vi "myRIO_BRig_FPGA_v3,31__PortC.vi"() -> ()   [LabVIEW 2014]
uses:
  <vilib>/rvi/FXPMathLib/FxpDiv/subVIs/nifxpmath_Div_SimConfig.ctl
  <vilib>/rvi/FXPMathLib/FxpSinAndCos/subVIs/nifxpmath_SinAndCos_SimConfig.ctl
  <vilib>/rvi/FXPMathLib/FxpDiv/simVIs/DllFxpDivTemp_sub.vi
  <vilib>/rvi/FXPMathLib/FxpSinAndCos/simVIs/DllFxpSinAndCosTemp_sub.vi
  <vilib>/rvi/Emulation/niFpgaGetClockAttributes.vi
  <vilib>/rvi/Emulation/niFpgaSctlEmulationGetInTimedLoop.vi
  <vilib>/rvi/Emulation/niFpgaEmulationReportErrorSimple.vi
  <vilib>/rvi/eio/common/nirviEmuTemplateMethod_errors.vi
  <vilib>/rvi/Emulation/niFpgaCriticalErrorInLSC.vi
  <vilib>/rvi/FXPMathLib/FxpDiv/XNode/nifxpmath_Div.xnode
  <vilib>/rvi/FXPMathLib/FxpMul/XNode/nifxpmath_Multiplier.xnode
  <vilib>/rvi/FXPMathLib/FxpSinAndCos/XNode/nifxpmath_SinAndCos.xnode
  <vilib>/rvi/FXPMathLib/FxpSub/XNode/nifxpmath_Sub.xnode
  <vilib>/eio/EIONode/EIONode.xnode
  <vilib>/rvi/FXPMathLib/sim/FxpSim.dll
panel:
  in  "laser_Nshutter":u32=100
  in  "AnaOut_0":i16
  in  "f_time_select":u32=173
  in  "laser_Nvalley":u32=100
  in  "laser_Npeak":u32=100
  in  "laserledMTrig":bool
  in  "tCycle_laser_wro":u32=100
  in  "tDelay_laser_wro":u32
  in  "tCycle_laser_rew":u32=100
  in  "tDelay_laser_rew":u32
  in  "laserResponse_reward_LED":bool
  in  "laserResponse_wrong_LED":bool
  out "SelectWrong":bool
  out "SelectReward":bool
  in  "laserResponse_wrong":bool
  in  "laserResponse_reward":bool
  in  "Left(F)_or_Right(T)":bool
  in  "ignoreWrong":bool
  in  "SelectionState":bool
  in  "laserMTrig":bool
  in  "FPGA_Stop":bool
  in  "audioTrigger_L":bool
  in  "audioTrigger_R":bool
  in  "audioFreq_L_Hz":u16=1000 min=1000 max=14000 step=1000
  in  "audioAmp_L":u16=1 min=1 max=32767 step=1
  in  "audioFreq_R_Hz":u16=1000 min=1000 max=14000 step=1000
  in  "audioAmp_R":u16=1 min=1 max=32767 step=1
  in  "A3_SL":bool
  in  "A1_SR":bool
  in  "Counts_Reset":bool
  out "A4_LickR":u32
  out "A2_LickL":u32
  in  "A6_Act":bool
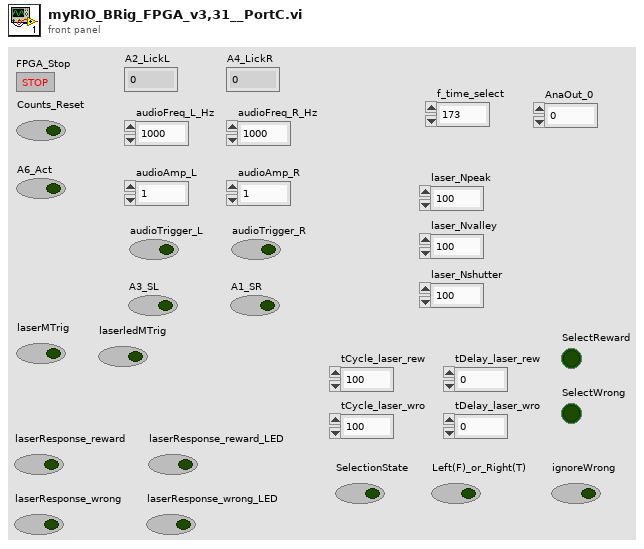
[diagram p1: front panel]
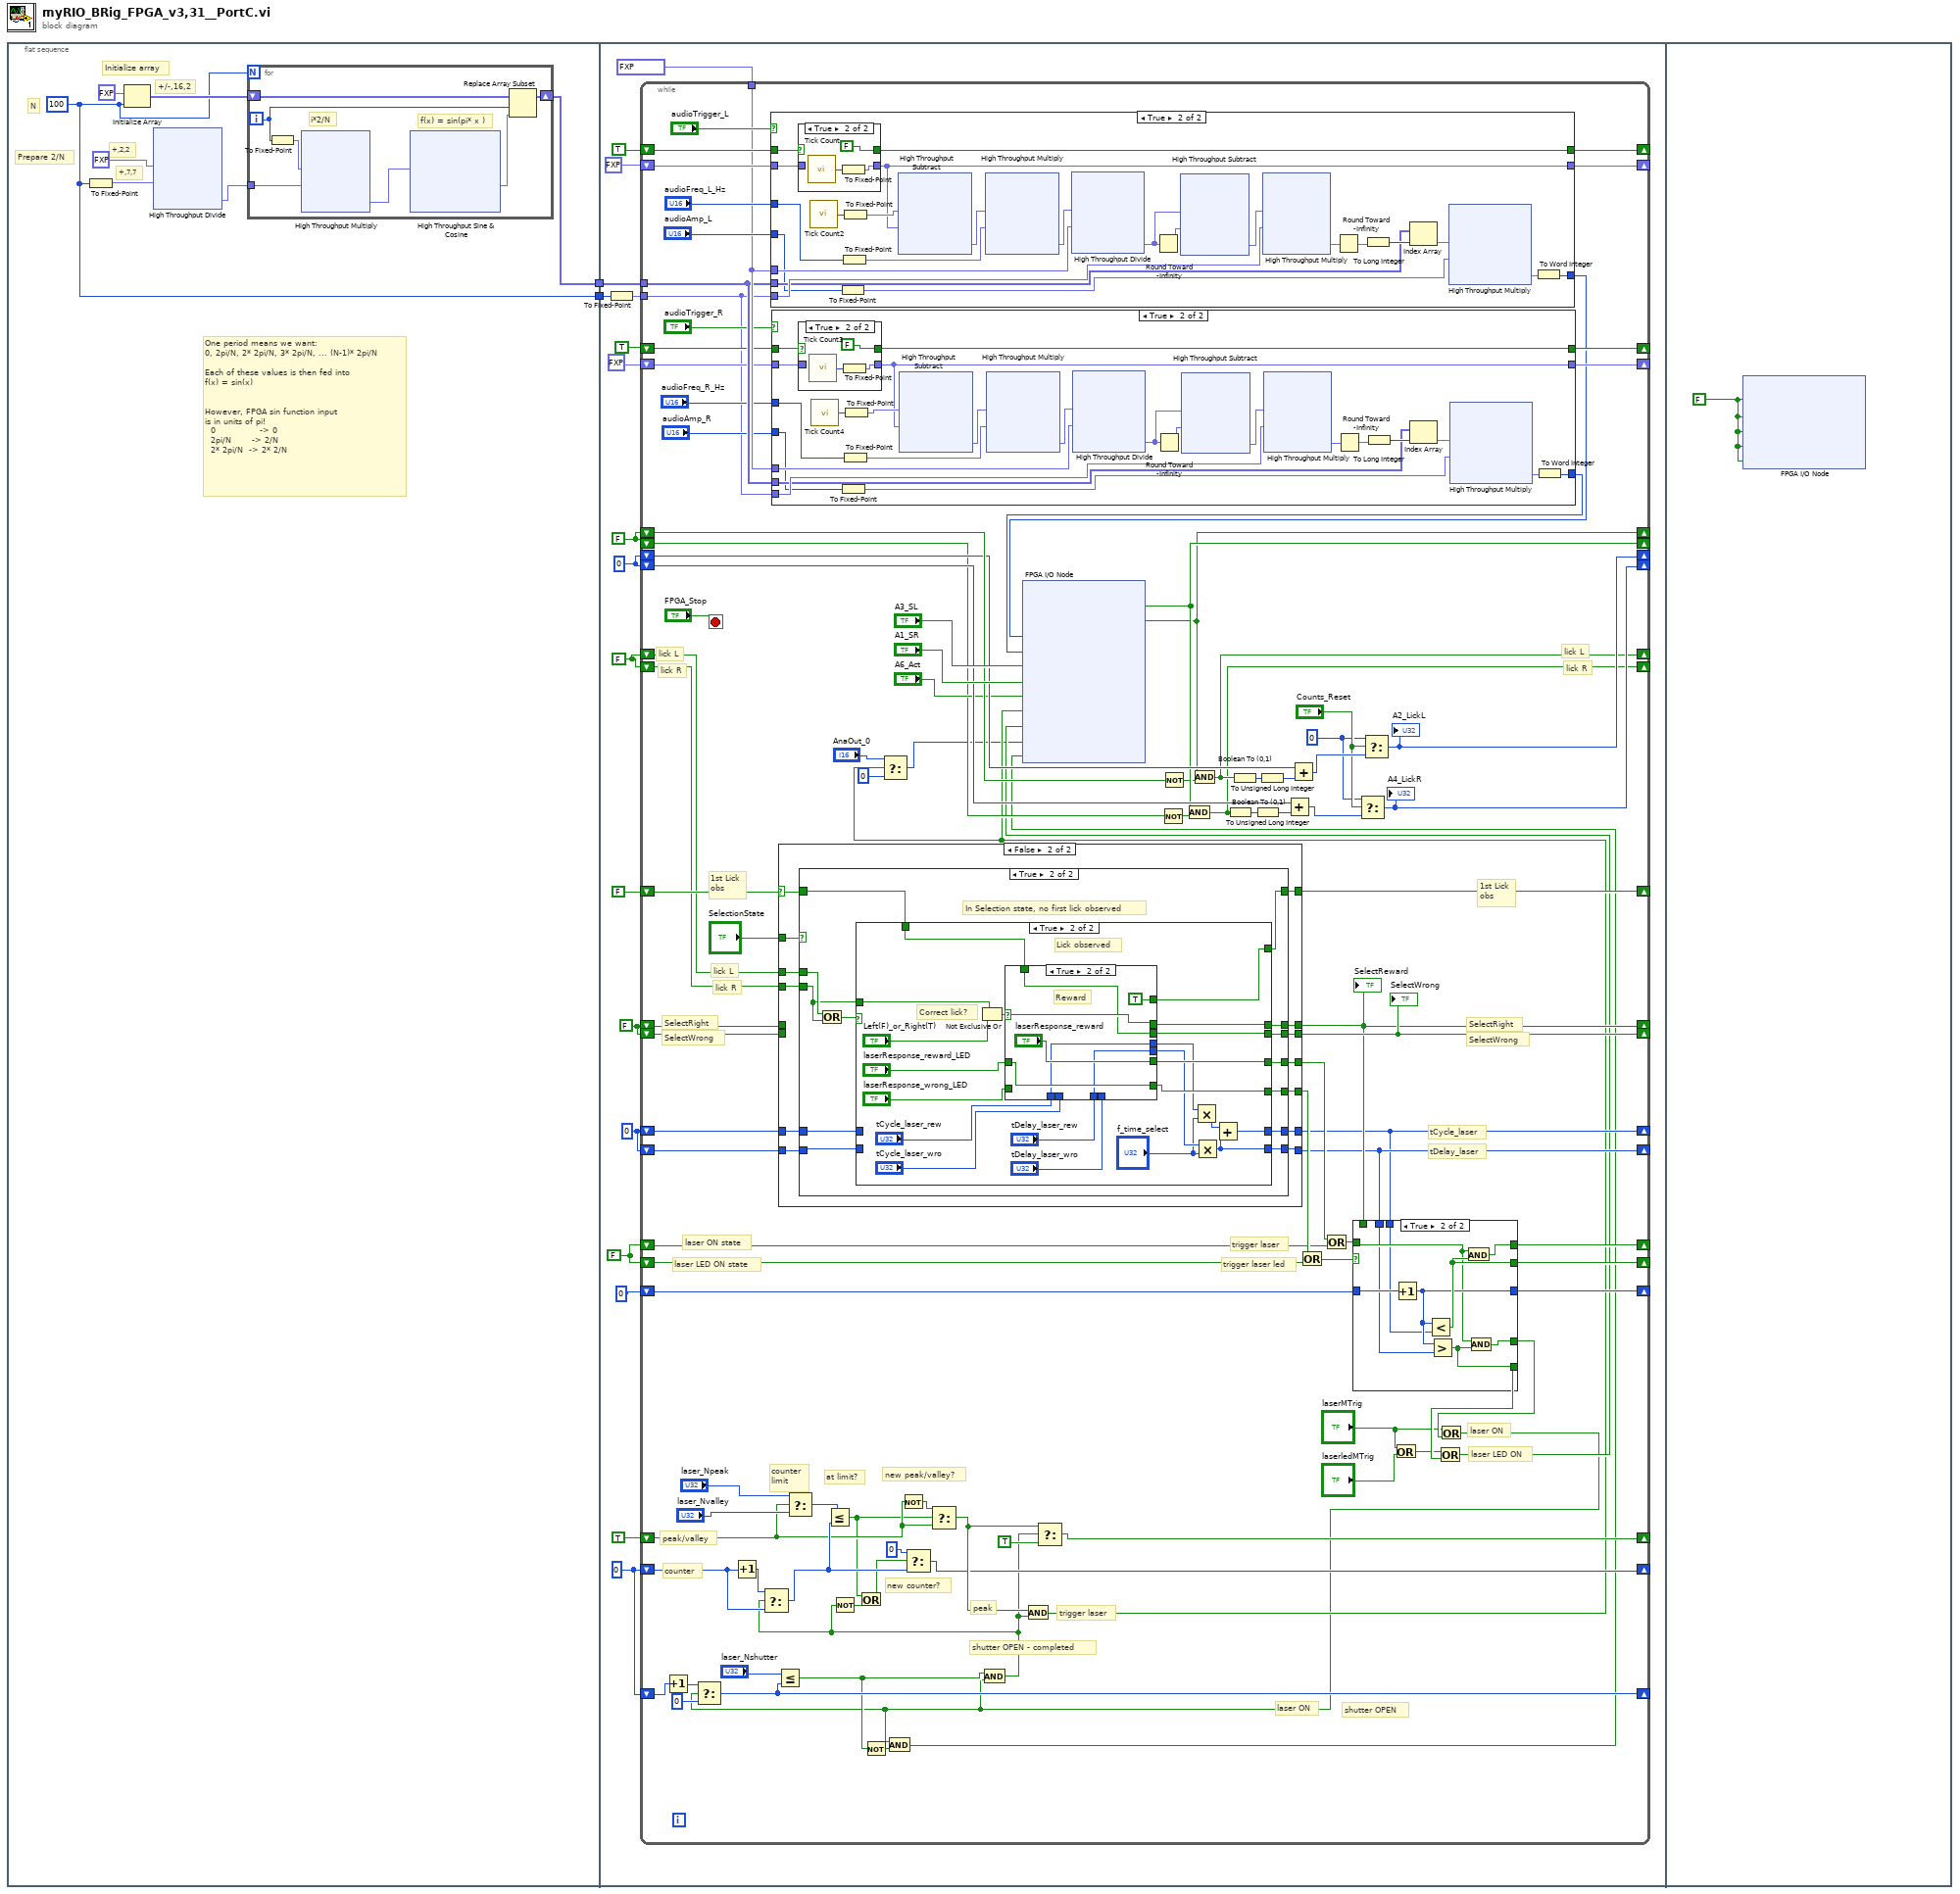
[diagram p0: block diagram]
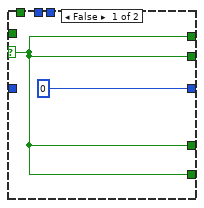
[diagram p2: hidden frame]
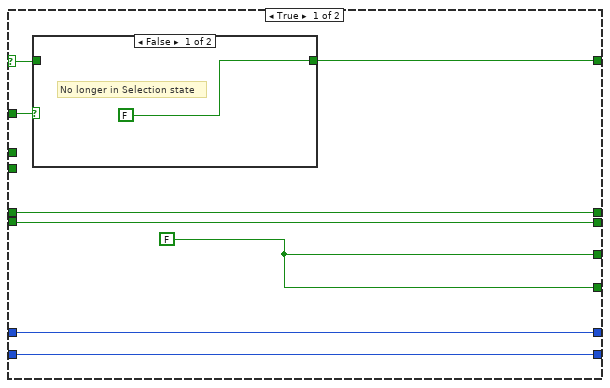
[diagram p3: hidden frame]
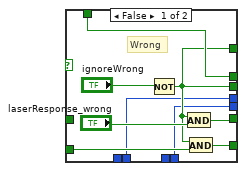
[diagram p7: hidden frame]
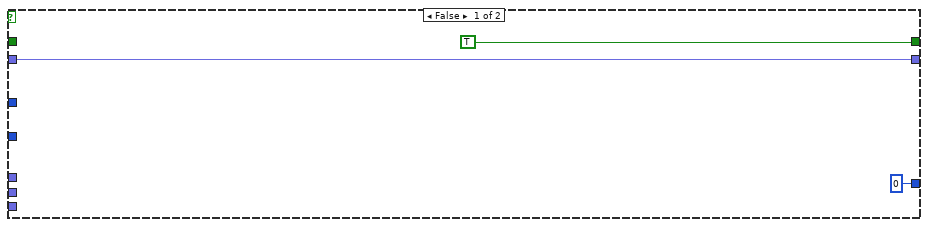
[diagram p8: hidden frame]
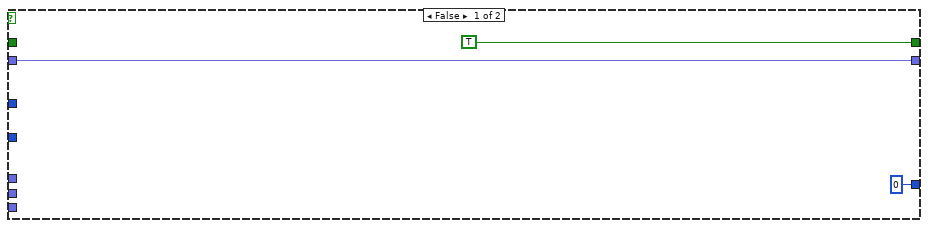
[diagram p10: hidden frame]
diagram:
  n1 = flat-sequence {
    tunnel: [w4] -> w2
    tunnel: [w3] -> w1
    tunnel: w2 -> [w86]
    tunnel: w1 -> [w88]
    frame #0 {
      w3 = 100 ("dimension size")
      # "N"
      # "+,7,7"
      # "+,2,2"
      # "+/-,16,2"
      # "Prepare 2/N"
      # "One period means we want:\n0, 2pi/N, 2* 2pi/N, 3* 2pi/N, ... (N-1)* 2pi/N\n\nEach of these values is then fed into\nf(x) = sin(x)\n\n\nHowever, FPGA sin function input\nis in units of pi!\n  0               -> 0\n  2pi/N       -> 2/N\n  2* 2pi/N  -> 2* 2/N"
      # "Initialize array"
      n2 = To Fixed-Point(number=w3) -> (fixed-point=w6:fxp<+,7,7>)  [unwired: 1 in]
      n3 = Initialize Array(fxp<+/-,16,2> 0.0 ("element"), w3) -> (w9:fxp<+/-,16,2>[])
      n4 = xnode "High Throughput Divide"("x"=fxp<+,2,2> 2.0, "y"=w6) -> ("x/y"=w5:fxp<+,27,0>)
      n5 = for {
        N: w3 -> [_]
        shift-right: [w42] -> w4
        shift-left: w9 -> [w43]
        tunnel: w5 -> [w38]
        i -> [w41]
        # "f(x) = sin(pi* x )"
        # "i*2/N"
        n6 = To Fixed-Point(number=w41) -> (fixed-point=w39:fxp<+,7,7>)  [unwired: 1 in]
        n7 = xnode ("High Throughput Multiply")("x"=w39, "y"=w38) -> ("x*y"=w37:fxp<+,34,7>)
        n8 = xnode "High Throughput Sine & Cosine"("x (pi)"=w37) -> ("sin(x)"=w40:fxp<+/-,16,2>)  [unwired: 1 out]
        n9 = Replace Array Subset(array=w43, new element=w40, index=w41) -> (w42:fxp<+/-,16,2>[])
      }
    }
    frame #1 {
      w74 = u32 0
      w76 = u32 0
      w78 = FALSE
      w77 = FALSE
      w81 = FALSE
      w82 = FALSE
      w83 = u32 0
      n10 = To Fixed-Point(number=w88) -> (fixed-point=w87:fxp<+,7,7>)  [unwired: 1 in]
      n11 = while {
        shift-right: [w187] -> _
        shift-left: TRUE -> [w191]
        shift-right: [w186] -> _
        shift-left: fxp<+,32,32> 0.0 -> [w190]
        tunnel: fxp<+,17,26> 40000000.0 -> [w185]
        tunnel: w87 -> [w178]
        tunnel: w86 -> [w184]
        shift-right: [w177] -> _
        shift-left: TRUE -> [w183]
        shift-right: [w176] -> _
        shift-left: fxp<+,32,32> 0.0 -> [w182]
        shift-right: [w153] -> _
        shift-left: w83 -> [w165]
        shift-right: [w156] -> _
        shift-left: w83 -> [w169]
        shift-right: [w157] -> _
        shift-left: w82 -> [w160]
        shift-right: [w154] -> _
        shift-left: w82 -> [w166]
        shift-right: [w151] -> _
        shift-left: FALSE -> [w150]
        shift-right: [w149] -> _
        shift-left: w81 -> [w147]
        shift-right: [w148] -> _
        shift-left: w81 -> [w146]
        shift-right: [w136] -> _
        shift-left: w77 -> [w138]
        shift-right: [w144] -> _
        shift-left: u32 0 -> [w145]
        shift-right: [w130] -> _
        shift-left: w78 -> [w142]
        shift-right: [w143] -> _
        shift-left: w78 -> [w141]
        shift-right: [w137] -> _
        shift-left: w77 -> [w134]
        shift-right: [w126] -> _
        shift-left: w76 -> [w129]
        shift-right: [w127] -> _
        shift-left: w76 -> [w128]
        shift-right: [w109] -> _
        shift-left: w74 -> [w120]
        shift-right: [w110] -> _
        shift-left: TRUE -> [w113]
        shift-right: [w97] -> _
        shift-left: w74 -> [w101]
        stop <- "FPGA_Stop" stop-if-true
        w162 = u32 0
        # "shutter OPEN"
        # "shutter OPEN - completed"
        # "trigger laser"
        # "peak"
        # "laser ON"
        # "new peak/valley?"
        # "counter"
        # "peak/valley"
        # "new counter?"
        # "at limit?"
        # "counter\nlimit"
        # "tDelay_laser"
        # "tCycle_laser"
        # "laser LED ON"
        # "laser ON"
        # "laser LED ON state"
        # "laser ON state"
        # "SelectWrong"
        # "SelectRight"
        # "SelectWrong"
        # "SelectRight"
        # "lick R"
        # "lick L"
        # "1st Lick\nobs"
        # "1st Lick\nobs"
        # "lick R"
        # "lick L"
        # "lick R"
        # "lick L"
        # "trigger laser led"
        # "trigger laser"
        n12 = Increment(x=w101) -> (x+1=w100:u32)
        n13 = Increment(x=w120) -> (x+1=w118:u32)
        n14 = case shown="True" "audioTrigger_L" {
          tunnel: w191 -> [_ w369]
          tunnel: w190 -> [w345 w368]
          tunnel: "audioFreq_L_Hz" -> [_ w365]
          tunnel: w185 -> [_ w362]
          tunnel: [w345 w346] -> w186
          tunnel: [TRUE w359] -> w187
          tunnel: w178 -> [_ w358]
          tunnel: w184 -> [_ w353]
          tunnel: "audioAmp_L" -> [_ w351]
          tunnel: [i16 0 w348] -> w172
          frame False {
          }
          frame True {
            n15 = case shown="True" w369 {
              selector: w369 -> [w398 _]
              tunnel: [w398 FALSE] -> w359
              tunnel: w368 -> [w397 _]
              tunnel: [w397 w399] -> w346
              frame False {
              }
              frame True {
                n16 = call "Tick Count"() -> ("Tick Count(Ticks)"=w401:u32)
                n17 = To Fixed-Point(number=w401) -> (fixed-point=w399:fxp<+,32,32>)  [unwired: 1 in]
              }
            }
            n18 = call "Tick Count2"() -> ("Tick Count(Ticks)"=w367:u32)
            n19 = To Fixed-Point(number=w351) -> (fixed-point=w350:fxp<+,15,15>)  [unwired: 1 in]
            n20 = To Fixed-Point(number=w365) -> (fixed-point=w364:fxp<+,14,14>)  [unwired: 1 in]
            n21 = To Fixed-Point(number=w367) -> (fixed-point=w347:fxp<+,32,32>)  [unwired: 1 in]
            n22 = xnode "High Throughput Subtract"("x"=w347, "y"=w346) -> ("x-y"=w366:fxp<+,32,32>)
            n23 = xnode ("High Throughput Multiply")("x"=w366, "y"=w364) -> ("x*y"=w363:fxp<+,46,46>)
            n24 = xnode "High Throughput Divide"("x"=w363, "y"=w362) -> ("x/y"=w361:fxp<+,34,21>)
            n25 = Round Toward -Infinity(1:w361) -> (0:w360:fxp<+,21,21>)
            n26 = xnode "High Throughput Subtract"("x"=w361, "y"=w360) -> ("x-y"=w357:fxp<+,14,1>)
            n27 = xnode ("High Throughput Multiply")("x"=w357, "y"=w358) -> ("x*y"=w354:fxp<+,21,8>)
            n28 = Round Toward -Infinity(1:w354) -> (0:w356:fxp<+,8,8>)
            n29 = To Long Integer(number=w356) -> (32bit integer=w355:i32)
            n30 = Index Array(array=w353, index=w355) -> (element=w352:fxp<+/-,16,2>)
            n31 = xnode ("High Throughput Multiply")("x"=w352, "y"=w350) -> ("x*y"=w349:fxp<+/-,31,17>)
            n32 = To Word Integer(number=w349) -> (16bit integer=w348:i16)
          }
        }
        n33 = case shown="True" "audioTrigger_R" {
          tunnel: w183 -> [_ w310]
          tunnel: w182 -> [w286 w309]
          tunnel: "audioFreq_R_Hz" -> [_ w306]
          tunnel: w185 -> [_ w303]
          tunnel: [w286 w287] -> w176
          tunnel: [TRUE w300] -> w177
          tunnel: w178 -> [_ w299]
          tunnel: w184 -> [_ w294]
          tunnel: "audioAmp_R" -> [_ w292]
          tunnel: [i16 0 w289] -> w173
          frame False {
          }
          frame True {
            n34 = case shown="True" w310 {
              selector: w310 -> [w339 _]
              tunnel: [w339 FALSE] -> w300
              tunnel: w309 -> [w338 _]
              tunnel: [w338 w340] -> w287
              frame False {
              }
              frame True {
                n35 = call "Tick Count3"() -> ("Tick Count(Ticks)"=w342:u32)
                n36 = To Fixed-Point(number=w342) -> (fixed-point=w340:fxp<+,32,32>)  [unwired: 1 in]
              }
            }
            n37 = call "Tick Count4"() -> ("Tick Count(Ticks)"=w308:u32)
            n38 = To Fixed-Point(number=w292) -> (fixed-point=w291:fxp<+,15,15>)  [unwired: 1 in]
            n39 = To Fixed-Point(number=w306) -> (fixed-point=w305:fxp<+,14,14>)  [unwired: 1 in]
            n40 = To Fixed-Point(number=w308) -> (fixed-point=w288:fxp<+,32,32>)  [unwired: 1 in]
            n41 = xnode "High Throughput Subtract"("x"=w288, "y"=w287) -> ("x-y"=w307:fxp<+,32,32>)
            n42 = xnode ("High Throughput Multiply")("x"=w307, "y"=w305) -> ("x*y"=w304:fxp<+,46,46>)
            n43 = xnode "High Throughput Divide"("x"=w304, "y"=w303) -> ("x/y"=w302:fxp<+,34,21>)
            n44 = Round Toward -Infinity(1:w302) -> (0:w301:fxp<+,21,21>)
            n45 = xnode "High Throughput Subtract"("x"=w302, "y"=w301) -> ("x-y"=w298:fxp<+,14,1>)
            n46 = xnode ("High Throughput Multiply")("x"=w298, "y"=w299) -> ("x*y"=w295:fxp<+,21,8>)
            n47 = Round Toward -Infinity(1:w295) -> (0:w297:fxp<+,8,8>)
            n48 = To Long Integer(number=w297) -> (32bit integer=w296:i32)
            n49 = Index Array(array=w294, index=w296) -> (element=w293:fxp<+/-,16,2>)
            n50 = xnode ("High Throughput Multiply")("x"=w293, "y"=w291) -> ("x*y"=w290:fxp<+/-,31,17>)
            n51 = To Word Integer(number=w290) -> (16bit integer=w289:i16)
          }
        }
        n52 = case shown="False" w150 {
          selector: w150 -> [w210 w225]
          tunnel: "SelectionState" -> [w212 w227]
          tunnel: [w211 w226] -> w151
          tunnel: w147 -> [_ w224]
          tunnel: w146 -> [_ w223]
          tunnel: [w209 w222] -> w135
          tunnel: [w207 w221] -> w130
          tunnel: [w208 w220] -> w143
          tunnel: w142 -> [w207 _]
          tunnel: w141 -> [w208 _]
          tunnel: [w209 w219] -> w139
          tunnel: [w206 w218] -> w126
          tunnel: [w205 w217] -> w127
          tunnel: w129 -> [w206 w216]
          tunnel: w128 -> [w205 w215]
          frame True {
            w209 = FALSE
            n53 = case shown="False" w212 {
              tunnel: [FALSE w214] -> w211
              tunnel: w210 -> [_ w214]
              frame False {
                # "No longer in Selection state"
              }
              frame True {
                # "Already observed first lick, no other action"
              }
            }
          }
          frame False {
            n54 = case shown="True" w227 {
              tunnel: [w230 w240] -> w226
              tunnel: w225 -> [w230 w236]
              tunnel: w224 -> [_ w242]
              tunnel: w223 -> [_ w241]
              tunnel: [w230 w239] -> w222
              tunnel: [w230 w238] -> w221
              tunnel: [w230 w237] -> w220
              tunnel: [w230 w235] -> w219
              tunnel: [w229 w234] -> w218
              tunnel: [w228 w233] -> w217
              tunnel: w216 -> [w229 w232]
              tunnel: w215 -> [w228 w231]
              frame False {
                # "Not in Selection state"
              }
              frame True {
                # "In Selection state, no first lick observed"
                n55 = Or(x=w242, y=w241) -> (x .or. y?=w243:bool)
                n56 = case shown="True" w243 {
                  tunnel: w241 -> [_ w266]
                  tunnel: [w246 w259] -> w240
                  tunnel: [w246 w264] -> w239
                  tunnel: [w246 w263] -> w238
                  tunnel: [w246 w262] -> w237
                  tunnel: w236 -> [w246 w261]
                  tunnel: [w246 w260] -> w235
                  tunnel: [w245 w248] -> w234
                  tunnel: [w244 w247] -> w233
                  tunnel: w232 -> [w245 _]
                  tunnel: w231 -> [w244 _]
                  frame False {
                  }
                  frame True {
                    # "Correct lick?"
                    # "Lick observed"
                    n57 = Not Exclusive Or(1:"Left(F)_or_Right(T)", 2:w266) -> (0:w265:bool)
                    n58 = case shown="True" w265 {
                      selector: w265 -> [_ w282]
                      tunnel: [w273 "laserResponse_reward"] -> w264
                      tunnel: [w271 w278] -> w262
                      tunnel: [w275 w282] -> w263
                      tunnel: w261 -> [w275 w278]
                      tunnel: [w272 w280] -> w260
                      tunnel: [w271 TRUE] -> w259
                      tunnel: "laserResponse_reward_LED" -> [_ w280]
                      tunnel: "laserResponse_wrong_LED" -> [w270 _]
                      tunnel: "tCycle_laser_rew" -> [_ w277]
                      tunnel: "tCycle_laser_wro" -> [w268 _]
                      tunnel: "tDelay_laser_rew" -> [_ w279]
                      tunnel: "tDelay_laser_wro" -> [w269 _]
                      tunnel: [w269 w279] -> w251
                      tunnel: [w268 w277] -> w250
                      frame False {
                        # "Wrong"
                        n59 = Not(x="ignoreWrong") -> (.not. x?=w271:bool)
                        n60 = And(x=w271, y="laserResponse_wrong") -> (x .and. y?=w273:bool)
                        n61 = And(x=w271, y=w270) -> (x .and. y?=w272:bool)
                      }
                      frame True {
                        # "Reward"
                      }
                    }
                    n62 = Multiply(x=w250, y="f_time_select") -> (x*y=w252:u32)
                    n63 = Multiply(x=w251, y="f_time_select") -> (x*y=w247:u32)
                    n64 = Add(x=w252, y=w247) -> (x+y=w248:u32)
                  }
                }
              }
            }
          }
        }
        "SelectWrong" <- w143
        "SelectReward" <- w130
        n65 = Select(t="laser_Npeak", s=w113, f="laser_Nvalley") -> (s? t:f=w122:u32)
        n66 = Not(x=w113) -> (.not. x?=w114:bool)
        n67 = Not(x=w160) -> (.not. x?=w159:bool)
        n68 = Not(x=w166) -> (.not. x?=w155:bool)
        n69 = Or(x=w139, y=w138) -> (x .or. y?=w140:bool)
        n70 = Or(x=w135, y=w134) -> (x .or. y?=w133:bool)
        n71 = case shown="True" w140 {
          selector: w140 -> [w194 _]
          tunnel: w145 -> [_ w204]
          tunnel: [u32 0 w201] -> w144
          tunnel: [w194 w202] -> w136
          tunnel: [w194 w203] -> w137
          tunnel: w133 -> [_ w200]
          tunnel: [w194 w199] -> w131
          tunnel: [w194 w198] -> w132
          tunnel: w130 -> [_ _]
          tunnel: w127 -> [_ w197]
          tunnel: w126 -> [_ w196]
          frame False {
          }
          frame True {
            n72 = Increment(x=w204) -> (x+1=w201:u32)
            n73 = Less?(x=w201, y=w196) -> (x < y?=w202:bool)
            n74 = Greater?(x=w201, y=w197) -> (0:w199:bool)
            n75 = And(x=w200, y=w202) -> (x .and. y?=w203:bool)
            n76 = And(x=w200, y=w199) -> (x .and. y?=w198:bool)
          }
        }
        n77 = Or(x="laserMTrig", y="laserledMTrig") -> (x .or. y?=w124:bool)
        n78 = Or(x=w124, y=w131) -> (x .or. y?=w119:bool)
        n79 = Or(x="laserMTrig", y=w132) -> (x .or. y?=w93:bool)
        n80 = Select(t=w100, s=w93, f=u32 0) -> (s? t:f=w97:u32)
        n81 = Less Or Equal?(x="laser_Nshutter", y=w97) -> (x <= y?=w95:bool)
        n82 = Not(x=w95) -> (.not. x?=w94:bool)
        n83 = And(x=w93, y=w94) -> (x .and. y?=w92:bool)
        n84 = And(x=w95, y=w93) -> (x .and. y?=w96:bool)
        n85 = Select(t=w118, s=w96, f=w120) -> (s? t:f=w117:u32)
        n86 = Less Or Equal?(x=w122, y=w117) -> (x <= y?=w107:bool)
        n87 = Not(x=w96) -> (.not. x?=w108:bool)
        n88 = Or(x=w107, y=w108) -> (x .or. y?=w106:bool)
        n89 = Select(t=u32 0, s=w106, f=w117) -> (s? t:f=w109:u32)
        n90 = Select(t=w114, s=w107, f=w113) -> (s? t:f=w112:bool)
        n91 = And(x=w112, y=w96) -> (x .and. y?=w105:bool)
        n92 = Select(t="AnaOut_0", s=w105, f=i16 0) -> (s? t:f=w104:i16)
        n93 = xnode "FPGA I/O Node"("AudioOut/Left"=w172, "AudioOut/Right"=w173, "ConnectorC/DIO3"="A3_SL", "ConnectorC/DIO1"="A1_SR", "ConnectorC/DIO6"="A6_Act", "ConnectorC/DIO0"=w105, "ConnectorC/DIO7"=w119, "ConnectorC/AO0"=w104, "ConnectorC/DIO5"=w92) -> ("ConnectorC/DIO4"=w157:bool, "ConnectorC/DIO2"=w154:bool)  [unwired: 11 in, 11 out]
        n94 = Select(t=w112, s=w96, f=TRUE) -> (s? t:f=w110:bool)
        n95 = And(x=w157, y=w159) -> (x .and. y?=w148:bool)
        n96 = And(x=w154, y=w155) -> (x .and. y?=w149:bool)
        n97 = Boolean To (0,1)(Boolean=w148) -> (0, 1=w171:i16)
        n98 = Boolean To (0,1)(Boolean=w149) -> (0, 1=w168:i16)
        n99 = To Unsigned Long Integer(number=w171) -> (unsigned 32bit integer=w170:u32)
        n100 = To Unsigned Long Integer(number=w168) -> (unsigned 32bit integer=w167:u32)
        n101 = Add(x=w169, y=w170) -> (x+y=w158:u32)
        n102 = Add(x=w165, y=w167) -> (x+y=w164:u32)
        n103 = Select(t=w162, s="Counts_Reset", f=w158) -> (s? t:f=w156:u32)
        "A4_LickR" <- w156
        n104 = Select(t=w162, s="Counts_Reset", f=w164) -> (s? t:f=w153:u32)
        "A2_LickL" <- w153
      }
    }
    frame #2 {
      w402 = FALSE ("ConnectorA/DIO3")
      n105 = xnode "FPGA I/O Node"("ConnectorC/DIO3"=w402, "ConnectorC/DIO1"=w402, "ConnectorC/DIO0"=w402, "ConnectorC/DIO6"=w402, "ConnectorC/DIO7"=w402) -> ()  [unwired: 5 in, 5 out]
    }
  }
